vi "Send Toggle Output.vi"(8 "error in":errorcluster, 11 "69X_79X in":refnum<class "6972A.lvclass">) -> (0 "error out":errorcluster, 3 "69X_79X out":refnum<class "6972A.lvclass">)   [LabVIEW 2019, in "6972A.lvlib" / "6972A.lvclass"]
uses:
  Library/6972A.lvclass
  C:/Users/Public/Documents/Development/builds/Instruments/PowerSupply.lvlibp/Library/PowerSupply.lvclass
  Accessors/Read Local Resource.vi
  Accessors/Write Local Resource.vi
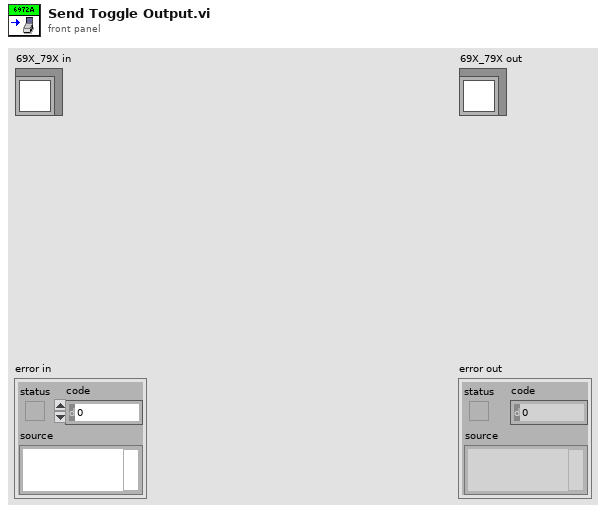
[diagram p1: front panel]
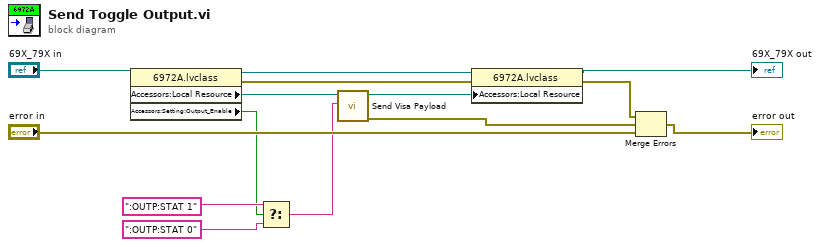
[diagram p0: block diagram]
diagram:
  n1 = property class="6972A.lvclass"(reference="69X_79X in") -> (reference out=w13:refnum<class "6972A.lvclass">, error out=w12:errorcluster, "Accessors:Local Resource"=w6:refnum<visa-resource-name>, "Accessors:Setting:Output_Enable"=w2:bool)  [unwired: 1 in]
  n2 = Select(t=":OUTP:STAT 1" ("write buffer"), s=w2, f=":OUTP:STAT 0" ("write buffer")) -> (s? t:f=w1:string)
  n3 = call "Send Visa Payload.vi"("Command"=w1, "Local Resource in"=w6) -> ("error out"=w5:errorcluster, "Local Resource out"=w7:refnum<visa-resource-name>)  [unwired: 8 in]
  n4 = property class="6972A.lvclass"(reference=w13, error in=w12, "Accessors:Local Resource"=w7) -> (reference out=→"69X_79X out":refnum<class "6972A.lvclass">, error out=w10:errorcluster)
  n5 = Merge Errors(w10, w5, "error in") -> (→"error out":errorcluster)
